vi "solar_voy Refnum SEQ to Voyager.vi"(1 "Voyager SEQ":refnum<queue>) -> (0 "Voyager Refnum":T1)   [LabVIEW 2018]
doc: "This type casts to the Voyager reference."
uses:
  solar_voy_ctl Voyager Refnum.ctl
  solar_voy_def/solar_voy_def_ctl PACKET_ID.ctl
  solar_voy_ctl Voyager.ctl
  solar_voy_def/solar_voy_def_ctl ITEM TYPE.ctl
  type/solar_type Item Type.ctl
  solar_voy_def/solar_voy_def_ctl ITEM.ctl
  solar_voy_def/solar_voy_def_ctl PACKET.ctl
  solar_voy_def/solar_voy_def_ctl HDR.ctl
  solar_voy_ctl TCP.ctl
  solar_voy_ctl Port Setup.ctl
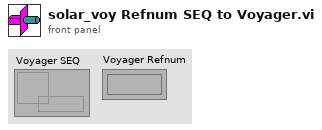
[diagram p1: front panel]
types:
  T1 = typedef "solar_voy_ctl Voyager Refnum.ctl" = refnum<k1>
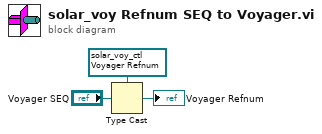
[diagram p0: block diagram]
diagram:
  w3 = T1 refnum items=["voyager"] ("Voyager Refnum 2")
  n1 = Type Cast(type=w3, x="Voyager SEQ") -> (*(type *) &x=→"Voyager Refnum":T1)
